vi "Modbus Slave.vi"   [LabVIEW 2016]
uses:
  <vilib>/Modbus/slave/Modbus Slave.lvclass
  <vilib>/Modbus/slave/Create Slave Instance (TCP).vi
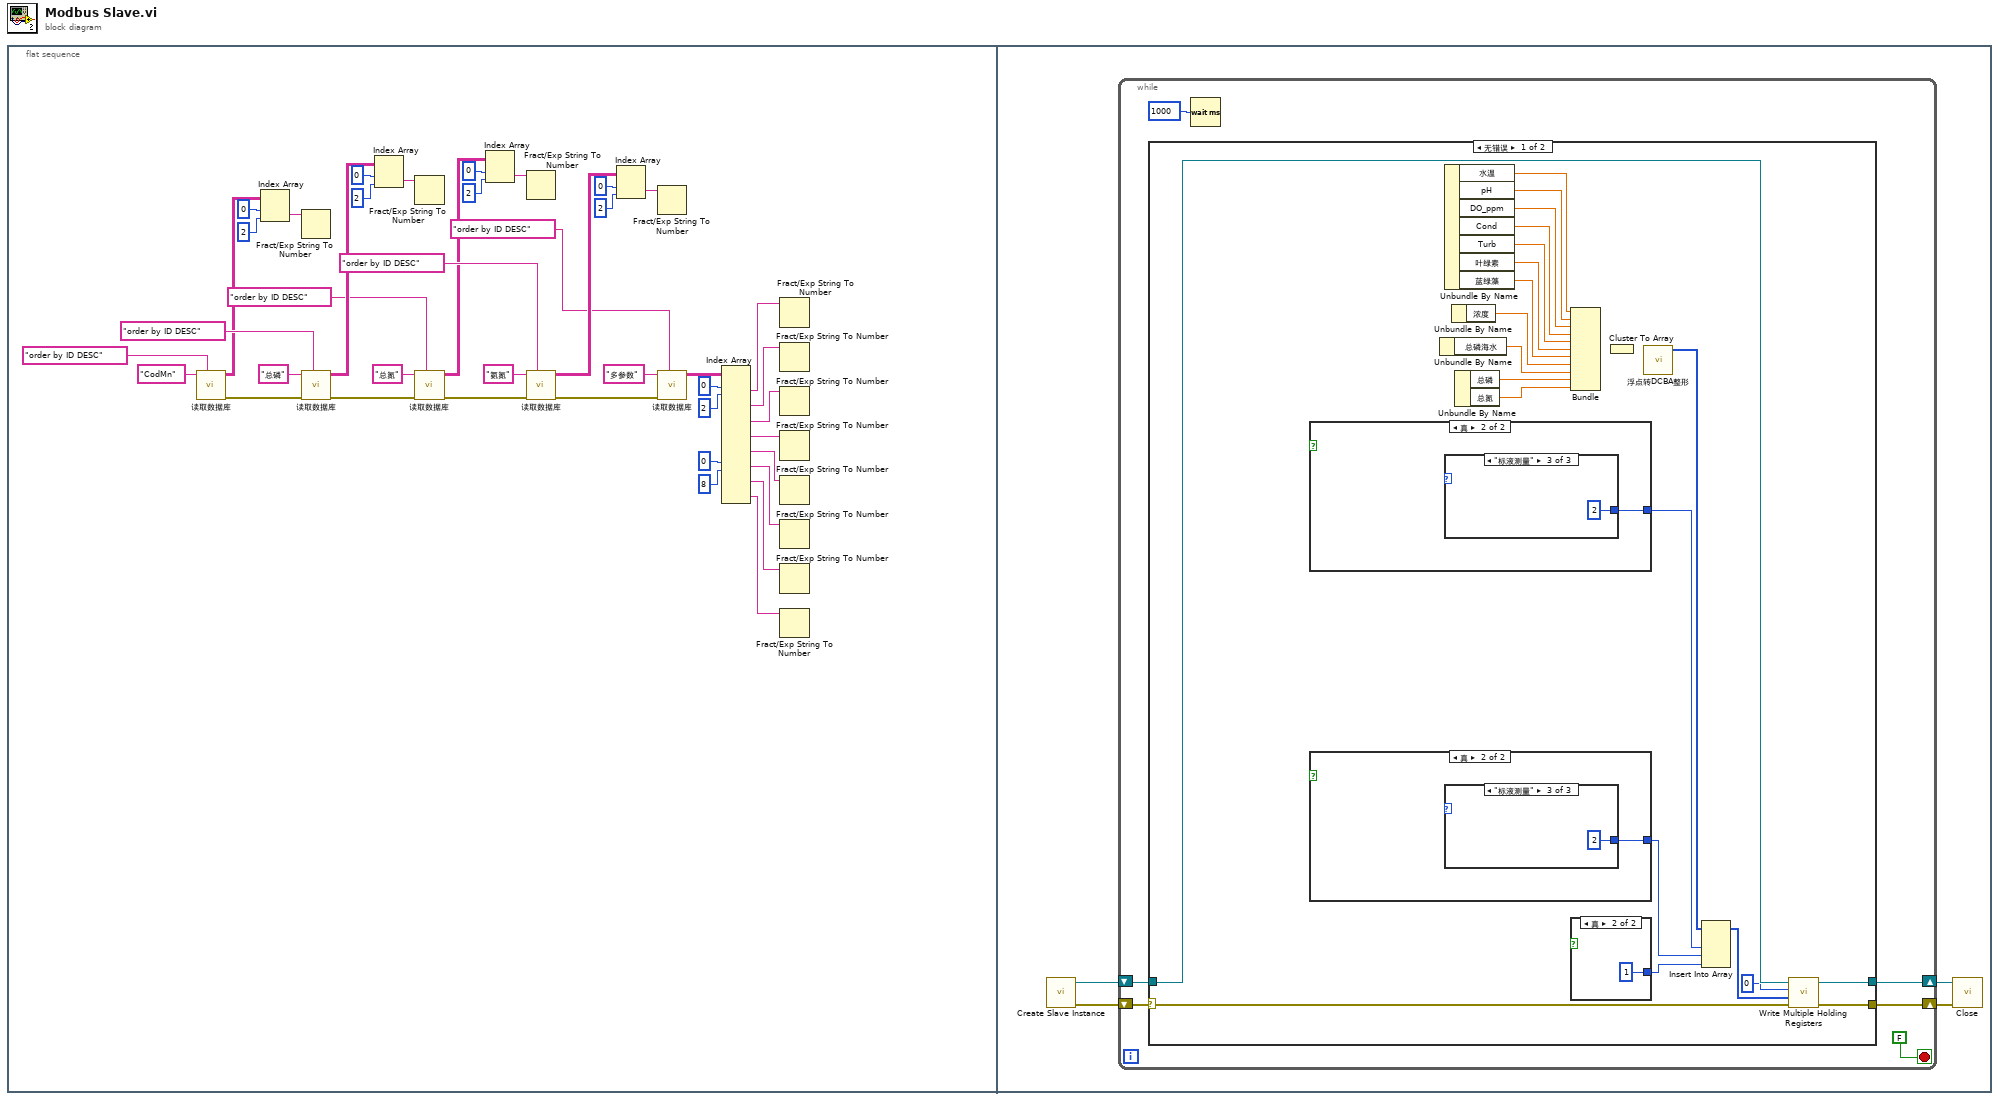
[diagram p0: block diagram]
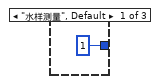
[diagram p4: hidden frame]
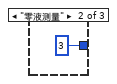
[diagram p5: hidden frame]
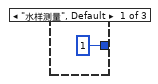
[diagram p7: hidden frame]
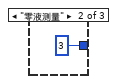
[diagram p8: hidden frame]
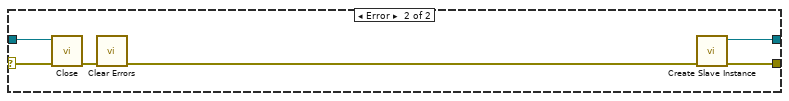
[diagram p9: hidden frame]
diagram:
  n1 = flat-sequence {
    frame #0 {
      n2 = call "读取数据库.vi"("condition"="order by ID DESC", "组合框"="CodMn" ("condition")) -> ("error out"=w4:errorcluster, "表格"=w25:string[][])  [unwired: 6 in, 2 out]
      n3 = Index Array(array=w25, index (row)=0 ("禁用的索引 (行)"), index (col)=2 ("禁用的索引 (列)")) -> (element=w24:string)
      n4 = Fract/Exp String To Number(string=w24) -> ()  [unwired: 3 in, 2 out]
      n5 = call "读取数据库.vi"("condition"="order by ID DESC", "error in (no error)"=w4, "组合框"="总磷" ("condition")) -> ("error out"=w3:errorcluster, "表格"=w32:string[][])  [unwired: 5 in, 2 out]
      n6 = Index Array(array=w32, index (row)=0 ("禁用的索引 (行)"), index (col)=2 ("禁用的索引 (列)")) -> (element=w35:string)
      n7 = Fract/Exp String To Number(string=w35) -> ()  [unwired: 3 in, 2 out]
      n8 = call "读取数据库.vi"("condition"="order by ID DESC", "error in (no error)"=w3, "组合框"="总氮" ("condition")) -> ("error out"=w2:errorcluster, "表格"=w26:string[][])  [unwired: 5 in, 2 out]
      n9 = Index Array(array=w26, index (row)=0 ("禁用的索引 (行)"), index (col)=2 ("禁用的索引 (列)")) -> (element=w27:string)
      n10 = Fract/Exp String To Number(string=w27) -> ()  [unwired: 3 in, 2 out]
      n11 = call "读取数据库.vi"("condition"="order by ID DESC", "error in (no error)"=w2, "组合框"="氨氮" ("condition")) -> ("error out"=w1:errorcluster, "表格"=w42:string[][])  [unwired: 5 in, 2 out]
      n12 = Index Array(array=w42, index (row)=0 ("禁用的索引 (行)"), index (col)=2 ("禁用的索引 (列)")) -> (element=w39:string)
      n13 = Fract/Exp String To Number(string=w39) -> ()  [unwired: 3 in, 2 out]
      n14 = call "读取数据库.vi"("condition"="order by ID DESC", "error in (no error)"=w1, "组合框"="多参数" ("condition")) -> ("表格"=w14:string[][])  [unwired: 5 in, 3 out]
      n15 = Index Array(array=w14, index (row) #1=0 ("禁用的索引 (行)"), index (col) #1=2 ("禁用的索引 (列)"), index (row) #6=0 ("禁用的索引 (行)"), index (col) #6=8 ("索引 (列)")) -> (element #1=w15:string, element #2=w13:string, element #3=w12:string, element #4=w11:string, element #5=w10:string, element #6=w7:string, element #7=w6:string, element #8=w5:string)  [unwired: 12 in]
      n16 = Fract/Exp String To Number(string=w15) -> ()  [unwired: 3 in, 2 out]
      n17 = Fract/Exp String To Number(string=w13) -> ()  [unwired: 3 in, 2 out]
      n18 = Fract/Exp String To Number(string=w12) -> ()  [unwired: 3 in, 2 out]
      n19 = Fract/Exp String To Number(string=w11) -> ()  [unwired: 3 in, 2 out]
      n20 = Fract/Exp String To Number(string=w10) -> ()  [unwired: 3 in, 2 out]
      n21 = Fract/Exp String To Number(string=w7) -> ()  [unwired: 3 in, 2 out]
      n22 = Fract/Exp String To Number(string=w6) -> ()  [unwired: 3 in, 2 out]
      n23 = Fract/Exp String To Number(string=w5) -> ()  [unwired: 3 in, 2 out]
    }
    frame #1 {
      n24 = call-poly <vilib>:"Create Slave Instance.vi"() -> ("error out"=w45:errorcluster, "TCP slave instance"=w44:refnum<class "Modbus Slave.lvclass">)  [unwired: 10 in]
      n25 = while {
        shift-right: [w52] -> w46
        shift-left: w44 -> [w53]
        shift-right: [w51] -> w47
        shift-left: w45 -> [w49]
        stop <- FALSE stop-if-true
        n26 = case shown="无错误" w49 {
          selector: w49 -> [w59 w86]
          tunnel: w53 -> [w74 w85]
          tunnel: [w73 w88] -> w52
          tunnel: [w72 w87] -> w51
          frame No Error {
            n27 = case shown="真" {
              selector: _ -> [_ _]
              tunnel: [_ w80] -> w56
              frame False {
              }
              frame True {
                n28 = case shown="\"标液测量\"" {
                  selector: _ -> [_ _ _]
                  tunnel: [1 3 2] -> w80
                  frame "水样测量", Default {
                  }
                  frame "零液测量" {
                  }
                  frame "标液测量" {
                  }
                }
              }
            }
            n29 = case shown="真" {
              selector: _ -> [_ _]
              tunnel: [_ w76] -> w55
              frame False {
              }
              frame True {
                n30 = case shown="\"标液测量\"" {
                  selector: _ -> [_ _ _]
                  tunnel: [1 3 2] -> w76
                  frame "水样测量", Default {
                  }
                  frame "零液测量" {
                  }
                  frame "标液测量" {
                  }
                }
              }
            }
            n31 = Unbundle By Name() -> ("总磷海水"=w62:sgl)  [unwired: 1 in]
            n32 = Unbundle By Name() -> ("水温"=w70:sgl, "pH"=w69:sgl, "DO_ppm"=w68:sgl, "Cond"=w67:sgl, "Turb"=w66:sgl, "叶绿素"=w65:sgl, "蓝绿藻"=w64:sgl)  [unwired: 1 in]
            n33 = Unbundle By Name() -> ("浓度"=w63:sgl)  [unwired: 1 in]
            n34 = Unbundle By Name() -> ("总磷"=w61:sgl, "总氮"=w60:sgl)  [unwired: 1 in]
            n35 = Bundle("水温"=w70, "pH"=w69, "DO_ppm"=w68, "Cond"=w67, "Turb"=w66, "叶绿素"=w65, "蓝绿藻"=w64, "浓度"=w63, "总磷海水"=w62, "总磷"=w61, "总氮"=w60) -> ()  [unwired: 1 in, 1 out]
            n36 = case shown="真" {
              selector: _ -> [_ _]
              tunnel: [_ 1] -> w54
              frame False {
              }
              frame True {
              }
            }
            n37 = Cluster To Array() -> ()  [unwired: 1 in, 1 out]
            n38 = call "浮点转DCBA整形.vi"() -> ("DCBA整形输出"=w58:u16[])  [unwired: 11 in]
            n39 = Insert Into Array(array=w58, new element #1=w56, new element #2=w55, new element #3=w54) -> (w57:u16[])  [unwired: 1 in]
            n40 = call-dynamic "Write Multiple Holding Registers.vi"("error in (no error)"=w59, "holding register values"=w57, "starting address"=u16 0, "Modbus slave in"=w74) -> ("error out"=w72:errorcluster, "Modbus slave out"=w73:refnum<class "Modbus Slave.lvclass">)  [unwired: 6 in]
          }
          frame Error {
            n41 = call-dynamic "Close.vi"("error in (no error)"=w86, "Modbus slave in"=w85) -> ("error out"=w84:errorcluster)  [unwired: 9 in]
            n42 = call <vilib>:"Clear Errors.vi"("error in (no error)"=w84) -> ("error out"=w89:errorcluster)  [unwired: 5 in, 1 out]
            n43 = call-poly <vilib>:"Create Slave Instance.vi"("error in (no error)"=w89) -> ("error out"=w87:errorcluster, "TCP slave instance"=w88:refnum<class "Modbus Slave.lvclass">)  [unwired: 9 in]
          }
        }
        n44 = Wait (ms)(milliseconds to wait=u32 1000 ("等待时间（毫秒）")) -> ()  [unwired: 1 out]
      }
      n45 = call-dynamic "Close.vi"("error in (no error)"=w47, "Modbus slave in"=w46) -> ()  [unwired: 9 in, 1 out]
    }
  }
